vi "niUSRP EX Tx Multiple Outputs (Single Device, Multi Channel).vi"() -> ()   [LabVIEW 2019]
doc: "Configures a single device to use two channels for transmission in a synchronous manner."
uses:
  <instrlib>/niUSRP/niUSRP Timestamp.ctl
  <instrlib>/niUSRP/niUSRP Configure Time Start Trigger.vi
  <instrlib>/niUSRP/niUSRP Write Tx Data (2D CDB).vi
  <vilib>/measure/NI_MABase.lvlib
panel:
  out "error out":errorcluster
  in  "Tab Control":enum32{"NI-294x/295x/X410", "NI-2900/2901"}(tab)
  in  "Channel 0 Carrier Frequency [Hz]":dbl=2000000000.0 format="%#_6p"
  in  "Channel 1 Carrier Frequency [Hz]":dbl=2000000000.0 format="%#_6p"
  in  "Carrier Frequency [Hz]":dbl=2000000000.0 format="%#_6p"
  in  "Start Trigger Time":T1={"whole seconds"=1, "fractional seconds"=0.0}
  in  "Channel 1 Active Antenna":string="TX1"
  in  "Channel 0 Active Antenna":string="TX1"
  in  "Channel 0 Tone Amplitude":dbl=0.7 step=0.05 format="%#.6g"
  in  "Channel 1 Tone Amplitude":dbl=0.4 step=0.05
  in  "Channel 1 Tone Frequency":dbl=15000.0 format="%#_6p"
  in  "Channel 0 Tone Frequency":dbl=10000.0 format="%#_6p"
  in  "Channel 1 Gain":dbl=10.0 format="%#_6f"
  in  "Stop":bool
  in  "Device Name":refnum<k15>="192.168.10.2"
  in  "Timeout":dbl=10.0
  in  "Number of Samples \nPer Write":i64=10000
  out "Waveform Graph":waveform(dbl)[](graph)
  in  "Channel 0 Gain":dbl=10.0 format="%#_6f"
  in  "IQ Rate [S/sec]":dbl=1000000.0 format="%#_6p"
  # "For X410 use TX/RX0"
  # "For X410 use TX/RX0"
  # "Note that the NI-2900 and NI-2901 use a single LO for both Tx channels"
  # "Time is set to 0 right \nbefore calling\nWrite Tx Data"
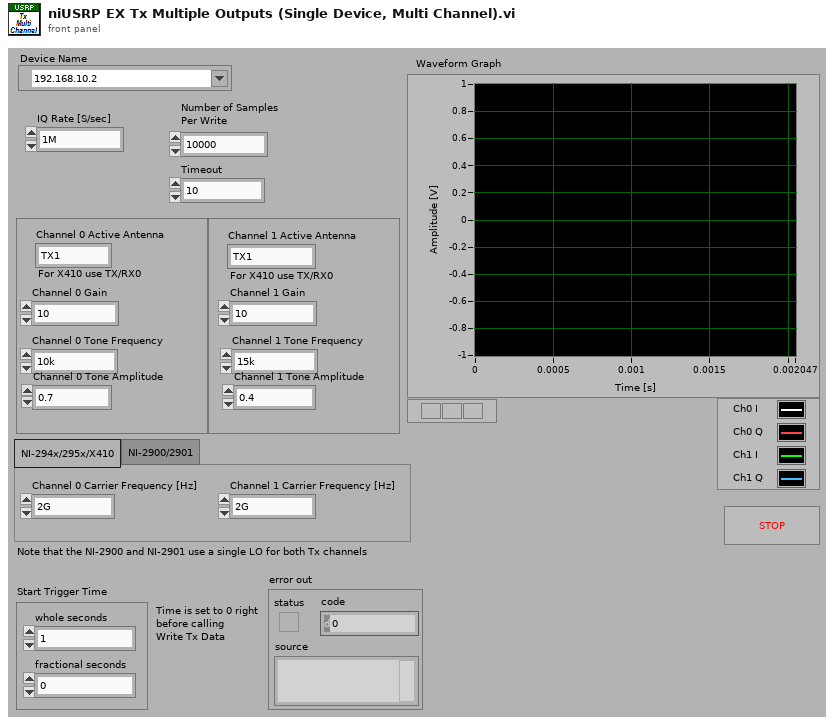
[diagram p1: front panel]
types:
  T1 = typedef "niUSRP Timestamp.ctl" = cluster{"whole seconds":u64, "fractional seconds":dbl}
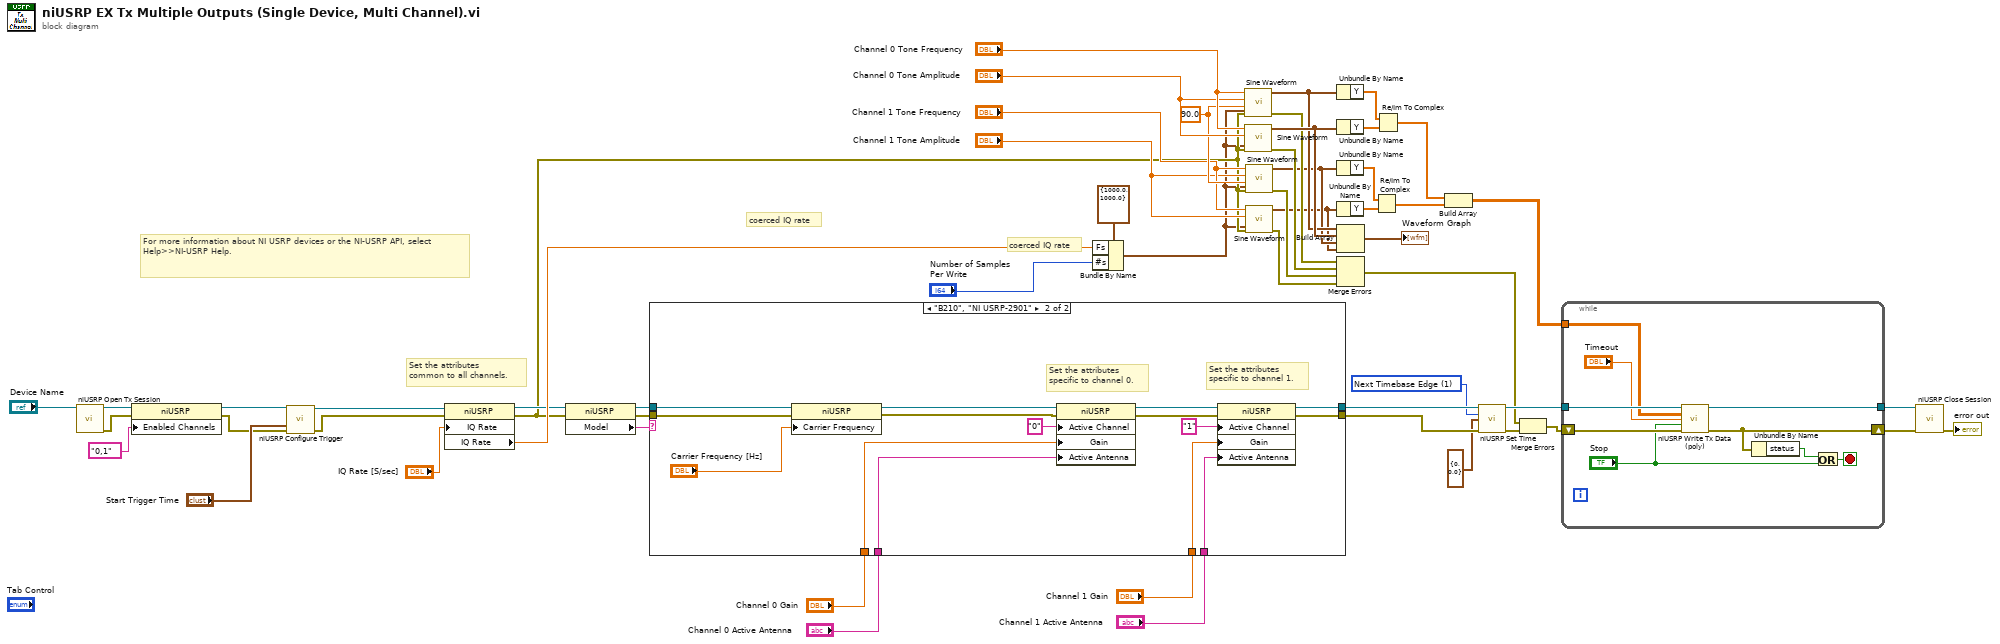
[diagram p0: block diagram]
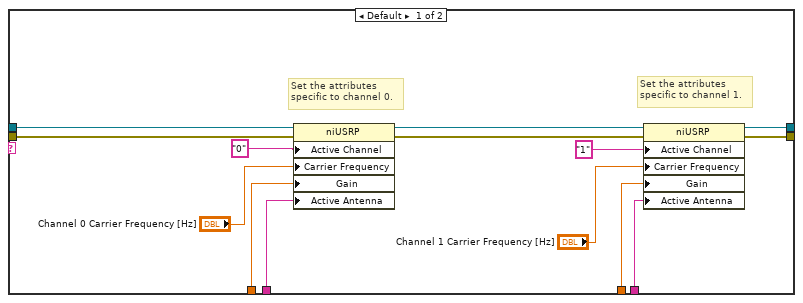
[diagram p2: hidden frame]
diagram:
  w26 = 1 items=["Now", "Next Timebase Edge"] ("apply timestamp")
  w9 = 90.0 ("phase")
  # "For more information about NI USRP devices or the NI-USRP API, select Help>>NI-USRP Help."
  # "coerced IQ rate"
  # "coerced IQ rate"
  # "Set the attributes\ncommon to all channels."
  n1 = call <instrlib>:"niUSRP Open Tx Session.vi"("device names"="Device Name") -> ("session handle out"=w25:refnum<k15>, "error out"=w24:errorcluster)  [unwired: 13 in]
  n2 = property class="niUSRP"(reference=w25, error in=w24, "Enabled Channels"="0,1" ("Configuration:Enabled Channels")) -> (reference out=w23:refnum<k15>, error out=w22:errorcluster)
  n3 = call-poly <instrlib>:"niUSRP Configure Trigger.vi"("session handle"=w23, "start trigger time"="Start Trigger Time", "error in (no error)"=w22) -> ("session handle out"=w21:refnum<k15>, "error out"=w20:errorcluster)  [unwired: 11 in]
  n4 = property class="niUSRP"(reference=w21, error in=w20, "IQ Rate"="IQ Rate [S/sec]") -> (reference out=w19:refnum<k15>, error out=w2:errorcluster, "IQ Rate"=w37:dbl)
  n5 = property class="niUSRP"(reference=w19, error in=w2) -> (reference out=w17:refnum<k15>, error out=w18:errorcluster, "Model"=w16:string)
  n6 = case shown="\"B210\", \"NI USRP-2901\"" w16 {
    tunnel: "Channel 0 Gain" -> [w69 w84]
    tunnel: "Channel 1 Gain" -> [w64 w79]
    tunnel: "Channel 0 Active Antenna" -> [w63 w78]
    tunnel: "Channel 1 Active Antenna" -> [w62 w77]
    tunnel: [w61 w76] -> w29
    tunnel: [w60 w75] -> w28
    tunnel: w18 -> [w59 w71]
    tunnel: w17 -> [w58 w74]
    frame Default {
      # "Set the attributes \nspecific to channel 1."
      # "Set the attributes \nspecific to channel 0."
      n7 = property class="niUSRP"(reference=w58, error in=w59, "Active Channel"="0", "Carrier Frequency"="Channel 0 Carrier Frequency [Hz]", "Gain"=w69, "Active Antenna"=w63) -> (reference out=w68:refnum<k15>, error out=w67:errorcluster)
      n8 = property class="niUSRP"(reference=w68, error in=w67, "Active Channel"="1", "Carrier Frequency"="Channel 1 Carrier Frequency [Hz]", "Gain"=w64, "Active Antenna"=w62) -> (reference out=w61:refnum<k15>, error out=w60:errorcluster)
    }
    frame "B210", "NI USRP-2901" {
      # "Set the attributes \nspecific to channel 1."
      # "Set the attributes \nspecific to channel 0."
      n9 = property class="niUSRP"(reference=w74, error in=w71, "Carrier Frequency"="Carrier Frequency [Hz]") -> (reference out=w73:refnum<k15>, error out=w72:errorcluster)
      n10 = property class="niUSRP"(reference=w73, error in=w72, "Active Channel"="0", "Gain"=w84, "Active Antenna"=w78) -> (reference out=w83:refnum<k15>, error out=w82:errorcluster)
      n11 = property class="niUSRP"(reference=w83, error in=w82, "Active Channel"="1", "Gain"=w79, "Active Antenna"=w77) -> (reference out=w76:refnum<k15>, error out=w75:errorcluster)
    }
  }
  n12 = Bundle By Name(cluster=cluster{"Fs":dbl, "#s":dbl} {"Fs"=1000.0, "#s"=1000.0} ("sampling info"), "Fs"=w37, "#s"="Number of Samples \nPer Write") -> (w1:cluster{"Fs":dbl, "#s":dbl})
  n13 = call <vilib>:"Sine Waveform.vi"("sampling info"=w1, "error in (no error)"=w2, "phase"=w9, "amplitude"="Channel 0 Tone Amplitude", "frequency"="Channel 0 Tone Frequency") -> ("error out"=w15:errorcluster, "signal out"=w49:waveform(dbl))  [unwired: 5 in]
  n14 = call <vilib>:"Sine Waveform.vi"("sampling info"=w1, "error in (no error)"=w2, "amplitude"="Channel 0 Tone Amplitude", "frequency"="Channel 0 Tone Frequency") -> ("error out"=w14:errorcluster, "signal out"=w50:waveform(dbl))  [unwired: 6 in]
  n15 = call <vilib>:"Sine Waveform.vi"("sampling info"=w1, "error in (no error)"=w2, "phase"=w9, "amplitude"="Channel 1 Tone Amplitude", "frequency"="Channel 1 Tone Frequency") -> ("error out"=w7:errorcluster, "signal out"=w8:waveform(dbl))  [unwired: 5 in]
  n16 = call <vilib>:"Sine Waveform.vi"("sampling info"=w1, "error in (no error)"=w2, "amplitude"="Channel 1 Tone Amplitude", "frequency"="Channel 1 Tone Frequency") -> ("error out"=w5:errorcluster, "signal out"=w6:waveform(dbl))  [unwired: 6 in]
  n17 = Unbundle By Name(w49) -> ("Y"=w48:dbl[])
  n18 = Unbundle By Name(w50) -> ("Y"=w47:dbl[])
  n19 = Unbundle By Name(w8) -> ("Y"=w44:dbl[])
  n20 = Unbundle By Name(w6) -> ("Y"=w45:dbl[])
  n21 = Build Array(w49, w50, w8, w6) -> (→"Waveform Graph":waveform(dbl)[])
  n22 = Merge Errors(w15, w14, w7, w5) -> (w11:errorcluster)
  n23 = Re/Im To Complex(1:w45, 2:w44) -> (0:w42:cdb[])
  n24 = Re/Im To Complex(1:w47, 2:w48) -> (0:w41:cdb[])
  n25 = Build Array(w41, w42) -> (w40:cdb[][])
  n26 = call <instrlib>:"niUSRP Set Time.vi"("session handle"=w29, "apply timestamp"=w26, "timestamp"=T1 {"whole seconds"=0, "fractional seconds"=0.0}, "error in (no error)"=w28) -> ("session handle out"=w30:refnum<k15>, "error out"=w13:errorcluster)  [unwired: 10 in]
  n27 = Merge Errors(w11, w13) -> (w12:errorcluster)
  n28 = while {
    tunnel: w30 -> [w93]
    tunnel: [w90] -> w39
    shift-right: [w89] -> w38
    shift-left: w12 -> [w92]
    tunnel: w40 -> [w86]
    stop <- w88 stop-if-true
    n29 = call-poly <instrlib>:"niUSRP Write Tx Data (poly).vi"("session handle"=w93, "data"=w86, "timeout"="Timeout", "end of data?"="Stop", "error in (no error)"=w92) -> ("session handle out"=w90:refnum<k15>, "error out"=w89:errorcluster)  [unwired: 9 in]
    n30 = Unbundle By Name(w89) -> ("status"=w87:bool)
    n31 = Or(x=w87, y="Stop") -> (x .or. y?=w88:bool)
  }
  n32 = call <instrlib>:"niUSRP Close Session.vi"("session handle"=w39, "error in (no error)"=w38) -> ("error out"=→"error out":errorcluster)  [unwired: 13 in]
